vi "correct_scanner_delay.vi"(0 "TrajectoryDL091126GenericVoxel in":refnum<class "TrajectoryDL091126GenericVoxel.lvclass">, 5 "x coordinates in":dbl[unit][](array[numeric]), 7 "y coordinates in":dbl[unit][](array[numeric]), 9 "z coordinates in":dbl[unit][](array[numeric]), 11 "error in (no error)":errorcluster) -> (4 "TrajectoryDL091126GenericVoxel out":refnum<class "TrajectoryDL091126GenericVoxel.lvclass">, 6 "x coordinates out":dbl[unit][](array[numeric]), 8 "y coordinates out":dbl[unit][](array[numeric]), 10 "z coordinates out":dbl[unit][](array[numeric]), 15 "error out":errorcluster)   [LabVIEW 2010, in "TrajectoryDL091126GenericVoxel.lvclass"]
uses:
  TrajectoryDL091126GenericVoxel.lvclass
  TrajectoryDL091126GenericVoxel.lvclass/TrajectoryDL091126GenericVoxel.ctl
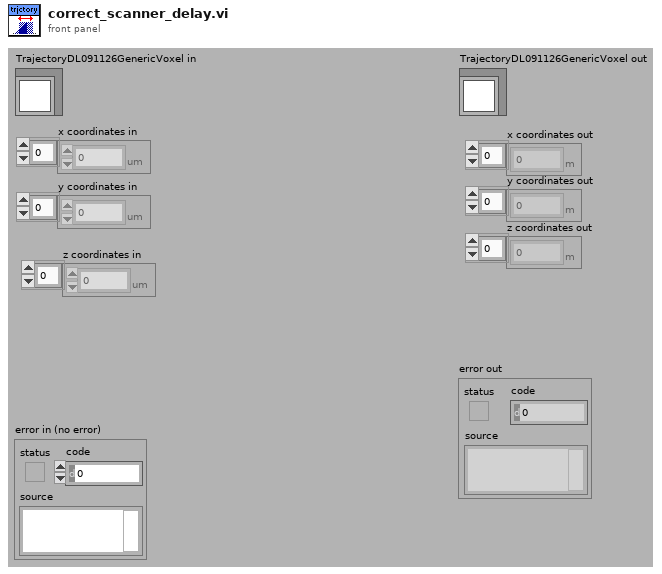
[diagram p1: front panel]
types:
  T1 = cluster{"scanner delays[0]":i32, "scanner delays[1]":i32, "scanner delays[2]":i32}
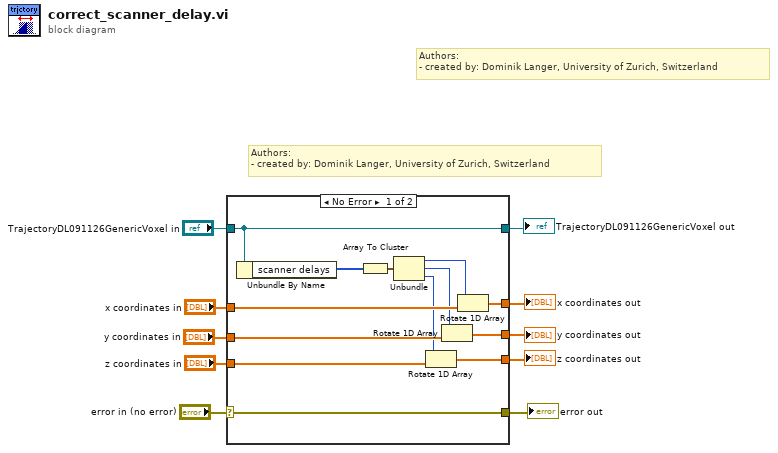
[diagram p0: block diagram]
diagram:
  # "Authors: \n- created by: Dominik Langer, University of Zurich, Switzerland"
  # "Authors: \n- created by: Dominik Langer, University of Zurich, Switzerland"
  n1 = case shown="No Error" "error in (no error)" {
    selector: "error in (no error)" -> [w19 w28]
    tunnel: [w19 w28] -> w4
    tunnel: [w12 w27] -> w1
    tunnel: "TrajectoryDL091126GenericVoxel in" -> [w12 w27]
    tunnel: "x coordinates in" -> [w23 w26]
    tunnel: "y coordinates in" -> [w17 w25]
    tunnel: "z coordinates in" -> [w18 w24]
    tunnel: [w22 w26] -> w7
    tunnel: [w21 w25] -> w6
    tunnel: [w20 w24] -> w5
    frame No Error {
      n2 = Unbundle By Name(w12) -> ("scanner delays"=w11:i32[])
      n3 = Array To Cluster(array=w11) -> (cluster=w16:T1)
      n4 = Unbundle(w16) -> ("scanner delays[0]"=w15:i32, "scanner delays[1]"=w14:i32, "scanner delays[2]"=w13:i32)
      n5 = Rotate 1D Array(1:w18, 2:w13) -> (0:w20:dbl[unit][])
      n6 = Rotate 1D Array(1:w17, 2:w14) -> (0:w21:dbl[unit][])
      n7 = Rotate 1D Array(1:w23, 2:w15) -> (0:w22:dbl[unit][])
    }
    frame Error {
    }
  }
  "error out" <- w4
  "TrajectoryDL091126GenericVoxel out" <- w1
  "x coordinates out" <- w7
  "y coordinates out" <- w6
  "z coordinates out" <- w5
